vi "daq_output.vi"(4 "INIT e.gate Configuration":T1 {"StartTime" format="%#.10f"; "dActTimeToSecondFactor" format="%#.10f"; "StartTimeToDayFactor" format="%#_10f"}, 6 "INIT mode":enum16{"online", "demo", "compile"}(ring), 7 "INIT? (F)":bool, 8 "error in (no error)":errorcluster, 9 "value":dbl, 10 "channel":string) -> (0 "error out":errorcluster)   [LabVIEW 2022 SP3]
uses:
  Program Files (x86)/National Instruments/LabVIEW 2022/instr.lib/Gantner Instruments/Ethernet/Gantner-Instruments HighSpeedPort.llb/e.gate Configuration.ctl
  Program Files (x86)/National Instruments/LabVIEW 2022/instr.lib/Gantner Instruments/Ethernet/Gantner-Instruments HighSpeedPort.llb/e.gate Channel Data.ctl
  Program Files (x86)/National Instruments/LabVIEW 2022/instr.lib/Gantner Instruments/Ethernet/Gantner-Instruments HighSpeedPort.llb/e.gate Data Type.ctl
  Program Files (x86)/National Instruments/LabVIEW 2022/instr.lib/Gantner Instruments/Ethernet/Gantner-Instruments HighSpeedPort.llb/e.gate Protocol Type.ctl
  Program Files (x86)/National Instruments/LabVIEW 2022/instr.lib/Gantner Instruments/Ethernet/Gantner-Instruments HighSpeedPort.llb/e.gate Module  Data.ctl
  Program Files (x86)/National Instruments/LabVIEW 2022/instr.lib/Gantner Instruments/Ethernet/Gantner-Instruments HighSpeedPort.llb/e.gateHSP_DLLhandle.ctl
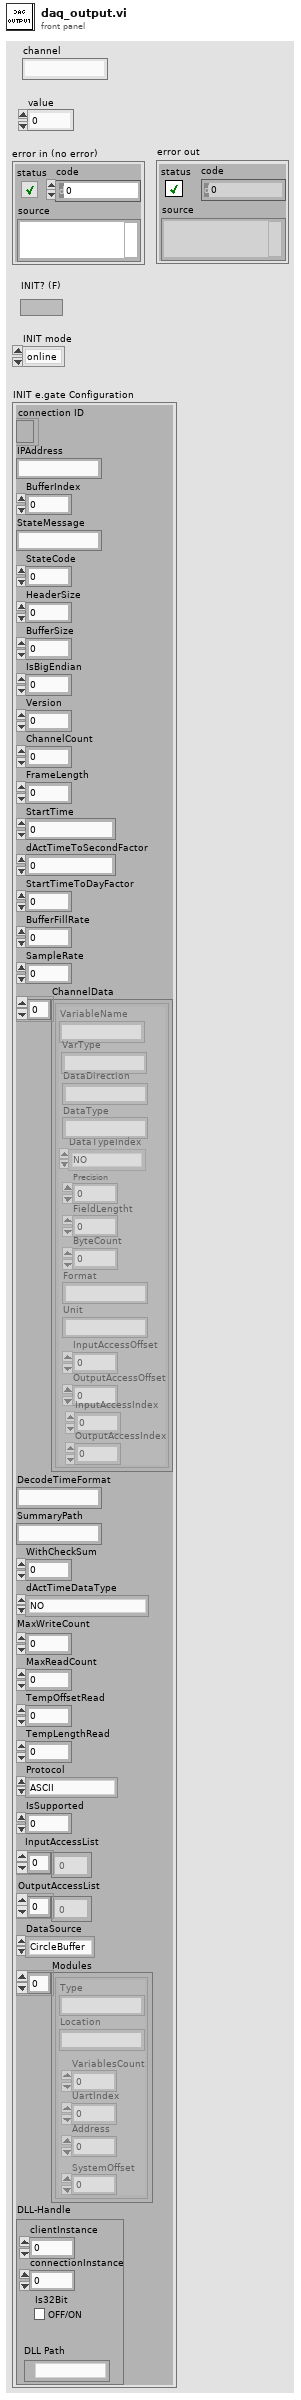
[diagram p1: front panel]
types:
  T1 = typedef "e.gate Configuration.ctl" = cluster{"connection ID":refnum<k5>, "IPAddress":string, "BufferIndex":i32, "StateMessage":string, "StateCode":i8, "HeaderSize":i32, "BufferSize":i32, "IsBigEndian":i32, "Version":i32, "ChannelCount":i32, "FrameLength":i32, "StartTime":dbl, "dActTimeToSecondFactor":dbl, "StartTimeToDayFactor":dbl, "BufferFillRate":dbl, "SampleRate":dbl, "ChannelData":T2[], "DecodeTimeFormat":string, "SummaryPath":string, "WithCheckSum":i32, "dActTimeDataType":T3, "MaxWriteCount":i32, "MaxReadCount":i32, "TempOffsetRead":i32, "TempLengthRead":i32, "Protocol":T4, "IsSupported":i32, "InputAccessList":i32[], "OutputAccessList":i32[], "DataSource":enum16{"CircleBuffer", "test.con Logger", "test.con Archive"}, "Modules":T5[], "DLL-Handle":T6}
  T2 = typedef "e.gate Channel Data.ctl" = cluster{"VariableName":string, "DataDirection":string, "DataType":string, "DataTypeIndex":T3, "Precision":i16, "FieldLengtht":i16, "ByteCount":i32, "Format":string, "Unit":string, "InputAccessOffset":i32, "OutputAccessOffset":i16, "InputAccessIndex":i16, "OutputAccessIndex":i16, "VarType":string}
  T3 = typedef "e.gate Data Type.ctl" = enum16{"NO", "BOOL", "SINT8", "USINT8", "SINT16", "USINT16", "SINT32", "USINT32", "FLOAT", "SET8", "SET16", "SET32", "DOUBLE", "SINT64", "USINT64", "SET64"}
  T4 = typedef "e.gate Protocol Type.ctl" = enum16{"ASCII", "HighspeedPort Online", "HighspeedPort Buffer (giutility.DLL) ", "PostProcessBuffer (giutility.DLL)"}
  T5 = typedef "e.gate Module  Data.ctl" = cluster{"Type":string, "Location":string, "VariablesCount":i16, "UartIndex":i16, "Address":i16, "SystemOffset":i16}
  T6 = typedef "e.gateHSP_DLLhandle.ctl" = cluster{"clientInstance":i32, "connectionInstance":i32, "Is32Bit":bool, "DLL Path":path}
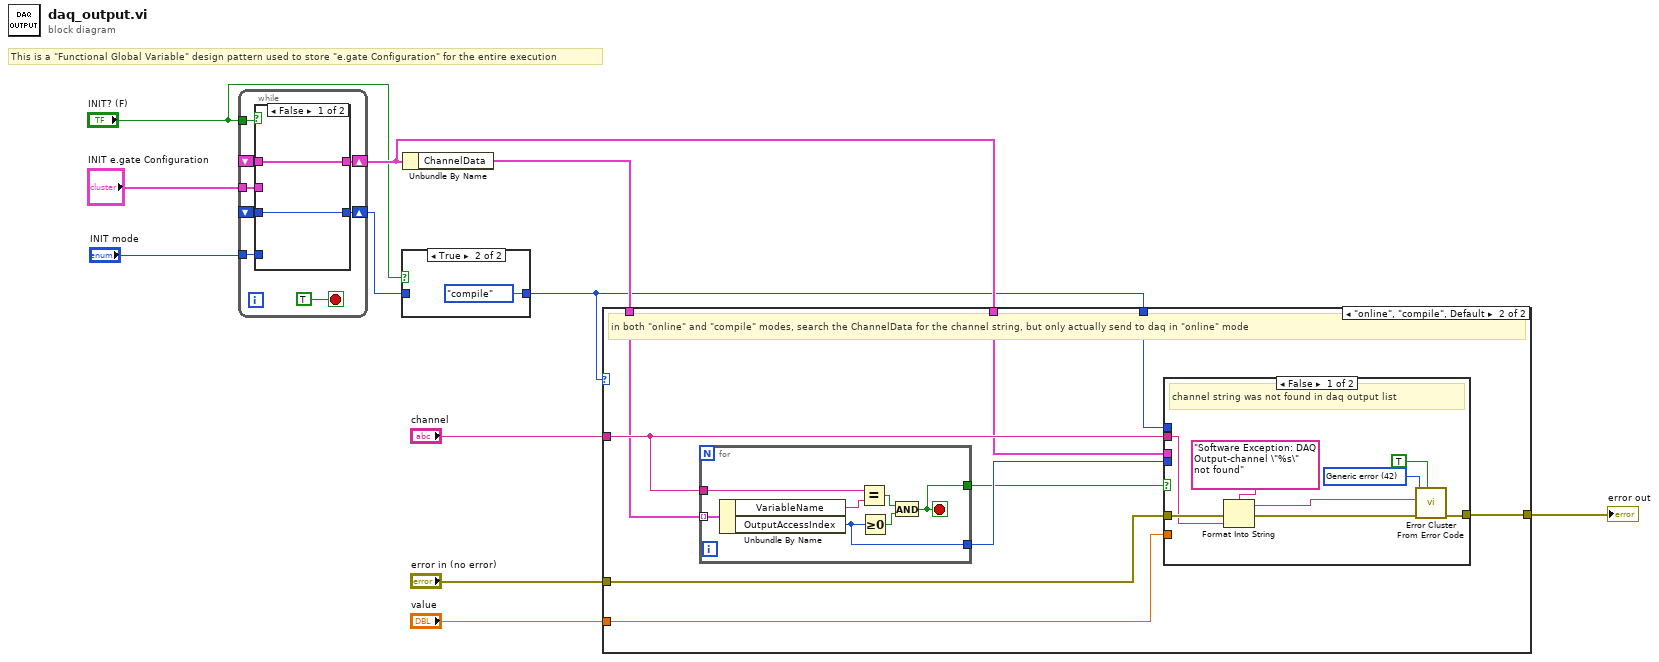
[diagram p0: block diagram]
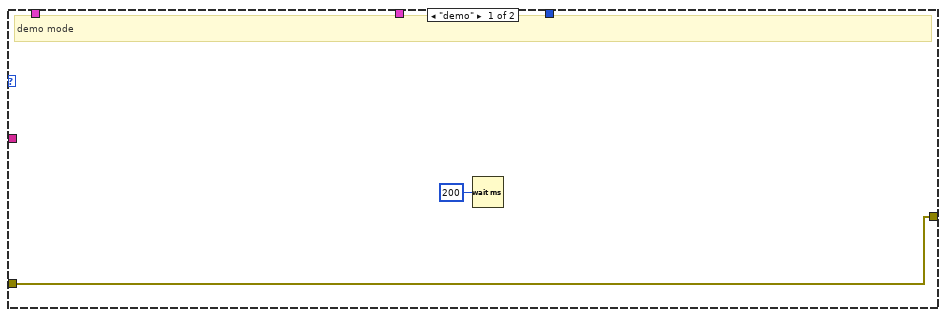
[diagram p2: hidden frame]
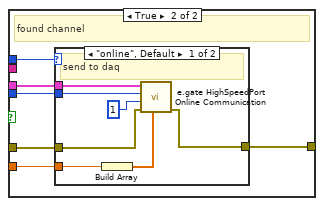
[diagram p3: hidden frame]
diagram:
  # "This is a \"Functional Global Variable\" design pattern used to store \"e.gate Configuration\" for the entire execution"
  n1 = while {
    tunnel: "INIT? (F)" -> [w18]
    shift-right: [w16] -> w6
    shift-left: _ -> [w15]
    tunnel: "INIT e.gate Configuration" -> [w17]
    shift-right: [w14] -> w3
    shift-left: _ -> [w12]
    tunnel: "INIT mode" -> [w13]
    stop <- TRUE stop-if-true
    n2 = case shown="False" w18 {
      tunnel: w17 -> [_ w23]
      tunnel: [w21 w23] -> w16
      tunnel: w15 -> [w21 _]
      tunnel: [w20 w22] -> w14
      tunnel: w13 -> [_ w22]
      tunnel: w12 -> [w20 _]
      frame False {
      }
      frame True {
      }
    }
  }
  n3 = case shown="True" "INIT? (F)" {
    tunnel: w3 -> [w24 _]
    tunnel: [w24 enum16{"online", "demo", "compile"}."compile" ("INIT mode")] -> w2
    frame False {
    }
    frame True {
    }
  }
  n4 = Unbundle By Name(w6) -> ("ChannelData"=w7:T2[])
  n5 = case shown="\"online\", \"compile\", Default" w2 {
    tunnel: "error in (no error)" -> [w27 w36]
    tunnel: "value" -> [_ w35]
    tunnel: "channel" -> [_ w34]
    tunnel: w7 -> [_ w33]
    tunnel: w6 -> [_ w32]
    tunnel: w2 -> [_ w31]
    tunnel: [w27 w28] -> w1
    frame "demo" {
      # "demo mode"
      n6 = Wait (ms)(milliseconds to wait=u32 200) -> ()  [unwired: 1 out]
    }
    frame "online", "compile", Default {
      # "in both \"online\" and \"compile\" modes, search the ChannelData for the channel string, but only actually send to daq in \"online\" mode"
      n7 = for {
        tunnel: w33 -> [w65] mode=indexing
        tunnel: [w61] -> w30
        tunnel: [w60] -> w29
        tunnel: w34 -> [w59]
        stop <- w60 stop-if-true
        n8 = Unbundle By Name(w65) -> ("VariableName"=w64:string, "OutputAccessIndex"=w61:i16)
        n9 = Equal?(x=w59, y=w64) -> (x = y?=w63:bool)
        n10 = Greater Or Equal To 0?(x=w61) -> (x >= 0?=w62:bool)
        n11 = And(x=w63, y=w62) -> (x .and. y?=w60:bool)
      }
      n12 = case shown="False" w29 {
        tunnel: w30 -> [_ w50]
        tunnel: w32 -> [_ w49]
        tunnel: w36 -> [w41 w48]
        tunnel: w35 -> [_ w47]
        tunnel: [w38 w46] -> w28
        tunnel: w34 -> [w40 _]
        tunnel: w31 -> [_ w45]
        frame False {
          w42 = 42 items=["No error", "Argument error", "Memory is full", "Out of zone", "End of file", "File already open", "Generic file I/O error", "File not found", "File permission error", "Disk is full", "Duplicate path", "Too many files open", "System feature not enabled", "Resource file not found", "Cannot add resource", "Resource not found", "Image not found", "Image memory error", "Pen does not exist", "Config type invalid", "Config token not found", "Config parse error", "Config memory error", "Bad external code format", "Bad external code offset", "External code not present", "Null window", "Destroy window error", "Null menu", "Print aborted", "Bad print record", "Print driver error", "Windows error during printing", "Memory error during printing", "Print dialog error", "Generic print error", "Invalid device refnum", "Device not found", "Device parameter error", "Device unit error", "Cannot open device", "Device call aborted", "Generic error", "Cancelled by user", "Object ID too low", "Object ID too high", "Object not in heap", "Unknown heap", "Unknown object (invalid DefProc)", "Unknown object (DefProc not in table)", "Message out of range", "Invalid (null) method", "Unknown message", "Manager call not supported", "Bad address", "Network operation in progress", "Network operation timed out", "Connection is busy", "Network attribute not supported", "Network error", "Address in use", "System out of memory", "Connection aborted", "Connection refused", "Not connected", "Already connected", "Connection closed", "Initialization error (interapplication manager)", "Bad occurrence", "Wait on unbound occurrence handler", "Occurrence queue overflow", "Datalog type conflict", "Unused", "Unrecognized type (interapplication manager)", "Memory corrupt", "Failed to make temporary DLL", "Old CIN version", "Drag socket not found", "Failed to load drop-object", "Failed to register OLE object", "Failed to release OLE object", "Format specifier type mismatch", "Unknown format specifier", "Too few format specifiers", "Too many format specifiers", "Scan failed", "Newer CIN version", "Error converting to variant", "Runtime menu error", "Password tampered", "Variant attribute not found", "Incompatible variant data type", "Event data is not available", "Event Store is not present", "Occurrence is not found", "Event Queue is not created", "Event info is not available", "Refnum passed is NULL", "Error retrieving Class GUID", "Error retrieving CoClass GUID", "Error retrieving TypeLib GUID.", "Bad built application magic bytes.", "Specific driver is different from the specific driver associated with the Logical Name.", "There is no session opened to the class driver.", "Max Error", "MAX - Error with config objects", "MAX - Error loading configuration", "MAX - Group not supported"]
          # "channel string was not found in daq output list"
          n13 = Format Into String(format string="Software Exception: DAQ Output-channel \"%s\" not found" ("message"), error in=w41, w40) -> (resulting string=w43:string, error out=w44:errorcluster)  [unwired: 1 in]
          n14 = call <vilib>:"Error Cluster From Error Code.vi"("show call chain? (False)"=TRUE, "error in (no error)"=w44, "error message (\"\")"=w43, "error code (0)"=w42) -> ("error out"=w38:errorcluster)  [unwired: 5 in]
        }
        frame True {
          # "found channel"
          n15 = case shown="\"online\", Default" w45 {
            tunnel: w50 -> [w57 _]
            tunnel: w49 -> [w56 _]
            tunnel: w48 -> [w55 w58]
            tunnel: w47 -> [w54 _]
            tunnel: [w52 w58] -> w46
            frame "online", Default {
              # "send to daq"
              n16 = Build Array(w54) -> (w53:dbl[])
              n17 = call "e.gate HighSpeedPort Online Communication.vi"("ValueArray"=w53, "error in (no error)"=w55, "WriteCount"=1, "WriteIndex"=w57, "e.gate Configuration In"=w56) -> ("error out"=w52:errorcluster)  [unwired: 4 in, 2 out]
            }
            frame "compile" {
              # "don't send anything"
            }
          }
        }
      }
    }
  }
  "error out" <- w1
